vi "TSC Material Panel Color Levels--constant.vi"() -> (2 "front panel color levels":string[](array[string]))   [LabVIEW 2021, in "Material SubVIs.lvlib"]
doc: "CONSTANT VI defines the constant value for the front panel color Levels that are shown in the right click menu and are used in color application.\n\n<b>Code Developed By:</b> +\nDaniel Coons +\nTechnology Service Corporation +\nwww.tsc.com/atcs"
uses:
  Material SubVIs.lvlib
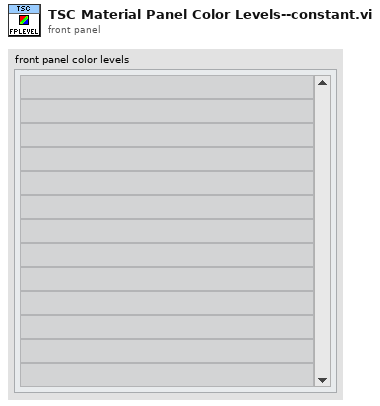
[diagram p1: front panel]
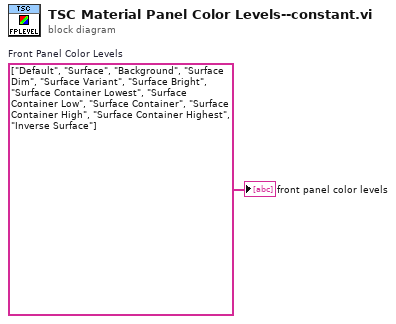
[diagram p0: block diagram]
diagram:
  w1 = string[] ["Default", "Surface", "Background", "Surface Dim", "Surface Variant", "Surface Bright", "Surface Container Lowest", "Surface Container Low", "Surface Container", "Surface Container High", "Surface Container Highest", "Inverse Surface"]  # Front Panel Color Levels
  "front panel color levels" <- w1
